vi "test_read-nmea-data2.vi"() -> ()   [LabVIEW 2019] (continued)
F9P\t\t\n15:11:02.15\tF9P\t\t\n15:11:02.17\tF9P\t\t\n15:11:02.19\tF9P\t\t\n15:11:02.21\tF9P\t\t\n15:11:02.23\tF9P\t\t\n15:11:02.25\tF9P\t$GNRMC,061104.00,A,3723.54880,N,12656.89488,E,2.304,137.20,250720,,,A,V*0F\n\t\n15:11:02.27\tF9P\t$GNVTG,137.20,T,,M,2.304,N,4.267,K,A*26\n\t\n15:11:02.29\tF9P\t$GNGGA,061104.00,3723.54880,N,12656.89488,E,1,12,0.68,63.8,M,18.5,M,,*7B\n\t\n15:11:02.31\tF9P\t$GNGSA,A,3,12,06,19,05,17,09,02,,,,,,1.28,0.68,1.08,1*08\n\t\n15:11:02.33\tF9P\t$GNGSA,A,3,85,71,84,,,,,,,,,,1.28,0.68,1.08,2*09\n\t\n15:11:02.35\tF9P\t$GNGSA,A,3,36,19,11,04,09,12,,,,,,,1.28,0.68,1.08,3*0C\n\t\n15:11:02.37\tF9P\t$GNGSA,A,3,14,11,33,,,,,,,,,,1.28,0.68,1.08,4*0D\n\t\n15:11:02.39\tF9P\t$GPGSV,3,1,09,02,54,318,32,04,18,044,,05,37,247,22,06,64,047,29,1*66\n\t\n15:11:02.41\tF9P\t$GPGSV,3,2,09,09,45,074,22,12,24,277,21,17,33,153,31,19,53,157,22,1*6D\n\t\n15:11:02.43\tF9P\t$GPGSV,3,3,09,25,12,307,,1*5D\n\t\n15:11:02.45\tF9P\t$GPGSV,3,1,09,02,54,318,,04,18,044,,05,37,247,,06,64,047,,6*6B\n\t\n15:11:02.47\tF9P\t$GPGSV,3,2,09,09,45,074,22,12,24,277,,17,33,153,13,19,53,157,,6*69\n\t\n15:11:02.49\tF9P\t$GPGSV,3,3,09,25,12,307,,6*5A\n\t\n15:11:02.51\tF9P\t$GLGSV,2,1,08,69,12,031,,70,72,041,,71,51,205,16,72,03,209,,1*75\n\t\n15:11:02.53\tF9P\t$GLGSV,2,2,08,77,01,326,,84,20,122,07,85,70,065,24,86,36,330,,1*7A\n\t\n15:11:02.55\tF9P\t$GLGSV,2,1,08,69,12,031,,70,72,041,,71,51,205,20,72,03,209,,3*72\n\t\n15:11:02.57\tF9P\t$GLGSV,2,2,08,77,01,326,,84,20,122,19,85,70,065,19,86,36,330,,3*79\n\t\n15:11:02.59\tF9P\t$GAGSV,2,1,08,02,08,297,10,04,66,118,24,09,31,193,18,11,71,357,20,7*79\n\t\n15:11:02.61\tF9P\t$GAGSV,2,2,08,12,40,102,19,19,27,045,09,25,09,249,,36,25,308,13,7*78\n\t\n15:11:02.63\tF9P\t$GAGSV,2,1,08,02,08,297,,04,66,118,25,09,31,193,,11,71,357,,2*77\n\t\n15:11:02.65\tF9P\t$GAGSV,2,2,08,12,40,102,27,19,27,045,,25,09,249,,36,25,308,,2*7B\n\t\n15:11:02.67\tF9P\t$GBGSV,1,1,03,11,50,131,19,14,87,138,20,33,60,219,22,1*45\n\t\n15:11:02.69\tF9P\t$GBGSV,1,1,03,11,50,131,29,14,87,138,21,33,60,219,,3*45\n\t\n15:11:02.71\tF9P\t$GNGLL,3723.54880,N,12656.89488,E,061104.00,A,A*72\n\t\n15:11:02.73\tF9P\t\t\n15:11:02.75\tF9P\t\t\n15:11:02.77\tF9P\t\t\n15:11:02.79\tF9P\t\t\n15:11:02.81\tF9P\t\t\n15:11:02.83\tF9P\t\t\n15:11:02.85\tF9P\t\t\n15:11:02.87\tF9P\t\t\n15:11:02.89\tF9P\t\t\n15:11:02.91\tF9P\t\t\n15:11:02.93\tF9P\t\t\n15:11:02.95\tF9P\t\t\n15:11:02.97\tF9P\t\t\n15:11:02.99\tF9P\t\t\n15:11:03.01\tF9P\t\t\n15:11:03.03\tF9P\t\t\n15:11:03.05\tF9P\t\t\n15:11:03.07\tF9P\t\t\n15:11:03.09\tF9P\t\t\n15:11:03.11\tF9P\t\t\n15:11:03.13\tF9P\t\t\n15:11:03.15\tF9P\t\t\n15:11:03.17\tF9P\t\t\n15:11:03.19\tF9P\t\t\n15:11:03.21\tF9P\t\t\n15:11:03.23\tF9P\t\t\n15:11:03.25\tF9P\t$GNRMC,061105.00,A,3723.54859,N,12656.89546,E,2.284,,250720,,,A,V*19\n\t\n15:11:03.27\tF9P\t$GNVTG,,T,,M,2.284,N,4.231,K,A*35\n\t\n15:11:03.29\tF9P\t$GNGGA,061105.00,3723.54859,N,12656.89546,E,1,12,0.69,62.1,M,18.5,M,,*74\n\t\n15:11:03.31\tF9P\t$GNGSA,A,3,12,06,19,05,17,09,02,,,,,,1.28,0.69,1.08,1*09\n\t\n15:11:03.33\tF9P\t$GNGSA,A,3,85,71,84,,,,,,,,,,1.28,0.69,1.08,2*08\n\t\n15:11:03.35\tF9P\t$GNGSA,A,3,36,19,11,04,09,12,,,,,,,1.28,0.69,1.08,3*0D\n\t\n15:11:03.37\tF9P\t$GNGSA,A,3,14,11,33,,,,,,,,,,1.28,0.69,1.08,4*0C\n\t\n15:11:03.39\tF9P\t$GPGSV,3,1,09,02,54,318,35,04,18,044,,05,37,247,23,06,64,047,24,1*6D\n\t\n15:11:03.41\tF9P\t$GPGSV,3,2,09,09,45,074,24,12,24,277,20,17,33,153,25,19,53,157,22,1*6F\n\t\n15:11:03.43\tF9P\t$GPGSV,3,3,09,25,12,307,,1*5D\n\t\n15:11:03.45\tF9P\t$GPGSV,3,1,09,02,54,318,,04,18,044,,05,37,247,,06,64,047,,6*6B\n\t\n15:11:03.47\tF9P\t$GPGSV,3,2,09,09,45,074,23,12,24,277,,17,33,153,17,19,53,157,,6*6C\n\t\n15:11:03.49\tF9P\t$GPGSV,3,3,09,25,12,307,,6*5A\n\t\n15:11:03.51\tF9P\t$GLGSV,2,1,08,69,12,031,,70,72,041,,71,51,205,16,72,03,209,,1*75\n\t\n15:11:03.53\tF9P\t$GLGSV,2,2,08,77,01,326,,84,20,122,10,85,70,065,24,86,36,330,,1*7C\n\t\n15:11:03.55\tF9P\t$GLGSV,2,1,08,69,12,031,,70,72,041,,71,51,205,20,72,03,209,,3*72\n\t\n15:11:03.57\tF9P\t$GLGSV,2,2,08,77,01,326,,84,20,122,20,85,70,065,19,86,36,330,,3*73\n\t\n15:11:03.59\tF9P\t$GAGSV,2,1,08,02,08,297,09,04,66,118,23,09,32,193,19,11,71,357,21,7*75\n\t\n15:11:03.61\tF9P\t$GAGSV,2,2,08,12,40,102,18,19,27,045,09,25,09,249,,36,25,308,15,7*7F\n\t\n15:11:03.63\tF9P\t$GAGSV,2,1,08,02,08,297,,04,66,118,24,09,32,193,,11,71,357,,2*75\n\t\n15:11:03.65\tF9P\t$GAGSV,2,2,08,12,40,102,26,19,27,045,,25,09,249,,36,25,308,,2*7A\n\t\n15:11:03.67\tF9P\t$GBGSV,1,1,03,11,50,131,18,14,87,138,22,33,60,219,22,1*46\n\t\n15:11:03.69\tF9P\t$GBGSV,1,1,03,11,50,131,25,14,87,138,21,33,60,219,,3*49\n\t\n15:11:03.71\tF9P\t$GNGLL,3723.54859,N,12656.89546,E,061105.00,A,A*74\n\t\n15:11:03.73\tF9P\t\t\n15:11:03.75\tF9P\t\t\n15:11:03.77\tF9P\t\t\n15:11:03.79\tF9P\t\t\n15:11:03.81\tF9P\t\t\n15:11:03.83\tF9P\t\t\n15:11:03.85\tF9P\t\t\n15:11:03.87\tF9P\t\t\n15:11:03.89\tF9P\t\t\n15:11:03.91\tF9P\t\t\n15:11:03.93\tF9P\t\t\n15:11:03.95\tF9P\t\t\n15:11:03.97\tF9P\t\t\n15:11:03.99\tF9P\t\t\n15:11:04.01\tF9P\t\t\n15:11:04.03\tF9P\t\t\n15:11:04.05\tF9P\t\t\n15:11:04.07\tF9P\t\t\n15:11:04.09\tF9P\t\t\n15:11:04.11\tF9P\t\t\n15:11:04.13\tF9P\t\t\n15:11:04.15\tF9P\t\t\n15:11:04.17\tF9P\t\t\n15:11:04.19\tF9P\t\t\n15:11:04.21\tF9P\t\t\n15:11:04.23\tF9P\t\t\n15:11:04.25\tF9P\t$GNRMC,061106.00,A,3723.54835,N,12656.89610,E,2.748,125.54,250720,,,A,V*0C\n\t\n15:11:04.27\tF9P\t$GNVTG,125.54,T,,M,2.748,N,5.089,K,A*29\n\t\n15:11:04.29\tF9P\t$GNGGA,061106.00,3723.54835,N,12656.89610,E,1,12,0.69,60.9,M,18.5,M,,*77\n\t\n15:11:04.31\tF9P\t$GNGSA,A,3,12,06,19,05,17,09,02,,,,,,1.28,0.69,1.08,1*09\n\t\n15:11:04.33\tF9P\t$GNGSA,A,3,85,71,84,,,,,,,,,,1.28,0.69,1.08,2*08\n\t\n15:11:04.35\tF9P\t$GNGSA,A,3,36,19,11,04,09,12,,,,,,,1.28,0.69,1.08,3*0D\n\t\n15:11:04.37\tF9P\t$GNGSA,A,3,14,11,33,,,,,,,,,,1.28,0.69,1.08,4*0C\n\t\n15:11:04.39\tF9P\t$GPGSV,3,1,09,02,54,318,36,04,18,044,,05,37,247,25,06,64,047,28,1*64\n\t\n15:11:04.41\tF9P\t$GPGSV,3,2,09,09,45,074,25,12,24,277,21,17,33,153,26,19,53,157,24,1*6A\n\t\n15:11:04.43\tF9P\t$GPGSV,3,3,09,25,12,307,,1*5D\n\t\n15:11:04.45\tF9P\t$GPGSV,3,1,09,02,54,318,,04,18,044,,05,37,247,,06,64,047,,6*6B\n\t\n15:11:04.47\tF9P\t$GPGSV,3,2,09,09,45,074,23,12,24,277,,17,33,153,18,19,53,157,,6*63\n\t\n15:11:04.49\tF9P\t$GPGSV,3,3,09,25,12,307,,6*5A\n\t\n15:11:04.51\tF9P\t$GLGSV,2,1,08,69,12,031,,70,72,041,,71,51,205,17,72,03,209,,1*74\n\t\n15:11:04.53\tF9P\t$GLGSV,2,2,08,77,01,326,,84,20,122,12,85,70,065,25,86,36,330,,1*7F\n\t\n15:11:04.55\tF9P\t$GLGSV,2,1,08,69,12,031,,70,72,041,,71,51,205,22,72,03,209,,3*70\n\t\n15:11:04.57\tF9P\t$GLGSV,2,2,08,77,01,326,,84,20,122,19,85,70,065,20,86,36,330,,3*73\n\t\n15:11:04.59\tF9P\t$GAGSV,2,1,08,02,08,297,07,04,66,118,25,09,32,193,18,11,71,358,22,7*70\n\t\n15:11:04.61\tF9P\t$GAGSV,2,2,08,12,40,102,18,19,27,045,11,25,09,249,,36,25,308,17,7*74\n\t\n15:11:04.63\tF9P\t$GAGSV,2,1,08,02,08,297,,04,66,118,23,09,32,193,,11,71,358,,2*7D\n\t\n15:11:04.65\tF9P\t$GAGSV,2,2,08,12,40,102,26,19,27,045,,25,09,249,,36,25,308,,2*7A\n\t\n15:11:04.67\tF9P\t$GBGSV,1,1,03,11,50,131,18,14,87,138,24,33,60,219,23,1*41\n\t\n15:11:04.69\tF9P\t$GBGSV,1,1,03,11,50,131,25,14,87,138,21,33,60,219,,3*49\n\t\n15:11:04.71\tF9P\t$GNGLL,3723.54835,N,12656.89610,E,061106.00,A,A*7D\n\t\n15:11:04.73\tF9P\t\t\n15:11:04.75\tF9P\t\t\n15:11:04.77\tF9P\t\t\n15:11:04.79\tF9P\t\t\n15:11:04.81\tF9P\t\t\n15:11:04.83\tF9P\t\t\n15:11:04.85\tF9P\t\t\n15:11:04.87\tF9P\t\t\n15:11:04.89\tF9P\t\t\n15:11:04.91\tF9P\t\t\n15:11:04.93\tF9P\t\t\n15:11:04.95\tF9P\t\t\n15:11:04.97\tF9P\t\t\n15:11:04.99\tF9P\t\t\n15:11:05.01\tF9P\t\t\n15:11:05.03\tF9P\t\t\n15:11:05.05\tF9P\t\t\n15:11:05.07\tF9P\t\t\n15:11:05.09\tF9P\t\t\n15:11:05.11\tF9P\t\t\n15:11:05.13\tF9P\t\t\n15:11:05.15\tF9P\t\t\n15:11:05.17\tF9P\t\t\n15:11:05.19\tF9P\t\t\n15:11:05.21\tF9P\t\t\n15:11:05.23\tF9P\t\t\n15:11:05.25\tF9P\t$GNRMC,061107.00,A,3723.54762,N,12656.89644,E,2.460,139.61,250720,,,A,V*03\n\t\n15:11:05.27\tF9P\t$GNVTG,139.61,T,,M,2.460,N,4.557,K,A*2C\n\t\n15:11:05.29\tF9P\t$GNGGA,061107.00,3723.54762,N,12656.89644,E,1,12,0.69,60.4,M,18.5,M,,*77\n\t\n15:11:05.31\tF9P\t$GNGSA,A,3,12,06,19,05,17,09,02,,,,,,1.28,0.69,1.08,1*09\n\t\n15:11:05.33\tF9P\t$GNGSA,A,3,85,71,84,,,,,,,,,,1.28,0.69,1.08,2*08\n\t\n15:11:05.35\tF9P\t$GNGSA,A,3,36,19,11,04,09,12,,,,,,,1.28,0.69,1.08,3*0D\n\t\n15:11:05.37\tF9P\t$GNGSA,A,3,14,11,33,,,,,,,,,,1.28,0.69,1.08,4*0C\n\t\n15:11:05.39\tF9P\t$GPGSV,3,1,09,02,54,318,28,04,18,044,,05,37,247,26,06,64,047,28,1*68\n\t\n15:11:05.41\tF9P\t$GPGSV,3,2,09,09,45,074,24,12,24,277,20,17,33,153,26,19,53,157,23,1*6D\n\t\n15:11:05.43\tF9P\t$GPGSV,3,3,09,25,12,307,,1*5D\n\t\n15:11:05.45\tF9P\t$GPGSV,3,1,09,02,54,318,,04,18,044,,05,37,247,,06,64,047,21,6*68\n\t\n15:11:05.47\tF9P\t$GPGSV,3,2,09,09,45,074,24,12,24,277,,17,33,153,18,19,53,157,,6*64\n\t\n15:11:05.49\tF9P\t$GPGSV,3,3,09,25,12,307,,6*5A\n\t\n15:11:05.51\tF9P\t$GLGSV,2,1,08,69,12,031,,70,72,041,,71,51,205,17,72,03,209,,1*74\n\t\n15:11:05.53\tF9P\t$GLGSV,2,2,08,77,01,326,,84,20,122,08,85,70,065,26,86,36,330,,1*77\n\t\n15:11:05.55\tF9P\t$GLGSV,2,1,08,69,12,031,,70,72,041,,71,51,205,21,72,03,209,,3*73\n\t\n15:11:05.57\tF9P\t$GLGSV,2,2,08,77,01,326,,84,20,122,20,85,70,065,21,86,36,330,,3*78\n\t\n15:11:05.59\tF9P\t$GAGSV,2,1,08,02,08,297,12,04,66,118,22,09,32,193,17,11,71,358,22,7*7C\n\t\n15:11:05.61\tF9P\t$GAGSV,2,2,08,12,40,102,17,19,27,045,13,25,09,249,,36,25,308,19,7*77\n\t\n15:11:05.63\tF9P\t$GAGSV,2,1,08,02,08,297,,04,66,118,21,09,32,193,,11,71,358,,2*7F\n\t\n15:11:05.65\tF9P\t$GAGSV,2,2,08,12,40,102,23,19,27,045,,25,09,249,,36,25,308,,2*7F\n\t\n15:11:05.67\tF9P\t$GBGSV,1,1,03,11,50,131,18,14,87,138,21,33,60,219,21,1*46\n\t\n15:11:05.69\tF9P\t$GBGSV,1,1,03,11,50,131,25,14,87,138,,33,60,219,,3*4A\n\t\n15:11:05.71\tF9P\t$GNGLL,3723.54762,N,12656.89644,E,061107.00,A,A*70\n\t\n15:11:05.73\tF9P\t\t\n15:11:05.75\tF9P\t\t\n15:11:05.77\tF9P\t\t\n15:11:05.79\tF9P\t\t\n15:11:05.81\tF9P\t\t\n15:11:05.83\tF9P\t\t\n15:11:05.85\tF9P\t\t\n15:11:05.87\tF9P\t\t\n15:11:05.89\tF9P\t\t\n15:11:05.91\tF9P\t\t\n15:11:05.93\tF9P\t\t\n15:11:05.95\tF9P\t\t\n15:11:05.97\tF9P\t\t\n15:11:05.99\tF9P\t\t\n15:11:06.01\tF9P\t\t\n15:11:06.03\tF9P\t\t\n15:11:06.05\tF9P\t\t\n15:11:06.07\tF9P\t\t\n15:11:06.09\tF9P\t\t\n15:11:06.11\tF9P\t\t\n15:11:06.13\tF9P\t\t\n15:11:06.15\tF9P\t\t\n15:11:06.17\tF9P\t\t\n15:11:06.19\tF9P\t\t\n15:11:06.21\tF9P\t\t\n15:11:06.23\tF9P\t\t\n15:11:06.25\tF9P\t$GNRMC,061108.00,A,3723.54695,N,12656.89698,E,3.008,136.67,250720,,,A,V*06\n\t\n15:11:06.27\tF9P\t$GNVTG,136.67,T,,M,3.008,N,5.572,K,A*28\n\t\n15:11:06.29\tF9P\t$GNGGA,061108.00,3723.54695,N,12656.89698,E,1,12,0.69,59.6,M,18.5,M,,*78\n\t\n15:11:06.31\tF9P\t$GNGSA,A,3,12,06,19,05,17,09,02,,,,,,1.28,0.69,1.08,1*09\n\t\n15:11:06.33\tF9P\t$GNGSA,A,3,85,71,84,,,,,,,,,,1.28,0.69,1.08,2*08\n\t\n15:11:06.35\tF9P\t$GNGSA,A,3,36,19,11,04,09,12,,,,,,,1.28,0.69,1.08,3*0D\n\t\n15:11:06.37\tF9P\t$GNGSA,A,3,14,11,33,,,,,,,,,,1.28,0.69,1.08,4*0C\n\t\n15:11:06.39\tF9P\t$GPGSV,3,1,09,02,54,318,34,04,18,044,15,05,37,247,25,06,64,047,30,1*6B\n\t\n15:11:06.41\tF9P\t$GPGSV,3,2,09,09,45,074,25,12,24,277,20,17,33,153,27,19,53,157,22,1*6C\n\t\n15:11:06.43\tF9P\t$GPGSV,3,3,09,25,12,307,,1*5D\n\t\n15:11:06.45\tF9P\t$GPGSV,3,1,09,02,54,318,,04,18,044,,05,37,247,20,06,64,047,21,6*6A\n\t\n15:11:06.47\tF9P\t$GPGSV,3,2,09,09,45,074,23,12,24,277,,17,33,153,18,19,53,157,,6*63\n\t\n15:11:06.49\tF9P\t$GPGSV,3,3,09,25,12,307,,6*5A\n\t\n15:11:06.51\tF9P\t$GLGSV,2,1,08,69,12,031,,70,72,041,,71,51,205,17,72,03,209,,1*74\n\t\n15:11:06.54\tF9P\t$GLGSV,2,2,08,77,01,326,,84,20,122,09,85,70,065,27,86,36,330,,1*77\n\t\n15:11:06.56\tF9P\t$GLGSV,2,1,08,69,12,031,,70,72,041,,71,51,205,21,72,03,209,,3*73\n\t\n15:11:06.58\tF9P\t$GLGSV,2,2,08,77,01,326,,84,20,122,19,85,70,065,23,86,36,330,,3*70\n\t\n15:11:06.60\tF9P\t$GAGSV,2,1,08,02,08,297,09,04,66,118,21,09,32,193,16,11,71,358,23,7*75\n\t\n15:11:06.62\tF9P\t$GAGSV,2,2,08,12,40,102,17,19,27,045,09,25,09,249,,36,25,308,18,7*7D\n\t\n15:11:06.64\tF9P\t$GAGSV,2,1,08,02,08,297,,04,66,118,23,09,32,193,,11,71,358,,2*7D\n\t\n15:11:06.66\tF9P\t$GAGSV,2,2,08,12,40,102,23,19,27,045,,25,09,249,,36,25,308,,2*7F\n\t\n15:11:06.68\tF9P\t$GBGSV,1,1,03,11,50,131,19,14,87,138,21,33,60,219,19,1*4C\n\t\n15:11:06.70\tF9P\t$GBGSV,1,1,03,11,50,131,31,14,87,138,,33,60,219,,3*4F\n\t\n15:11:06.72\tF9P\t$GNGLL,3723.54695,N,12656.89698,E,061108.00,A,A*77\n\t\n15:11:06.74\tF9P\t\t\n15:11:06.76\tF9P\t\t\n15:11:06.78\tF9P\t\t\n15:11:06.80\tF9P\t\t\n15:11:06.82\tF9P\t\t\n15:11:06.84\tF9P\t\t\n15:11:06.86\tF9P\t\t\n15:11:06.88\tF9P\t\t\n15:11:06.90\tF9P\t\t\n15:11:06.92\tF9P\t\t\n15:11:06.94\tF9P\t\t\n15:11:06.96\tF9P\t\t\n15:11:06.98\tF9P\t\t\n15:11:07.00\tF9P\t\t\n15:11:07.02\tF9P\t\t\n15:11:07.04\tF9P\t\t\n15:11:07.06\tF9P\t\t\n15:11:07.08\tF9P\t\t\n15:11:07.10\tF9P\t\t\n15:11:07.12\tF9P\t\t\n15:11:07.14\tF9P\t\t\n15:11:07.16\tF9P\t\t\n15:11:07.18\tF9P\t\t\n15:11:07.20\tF9P\t\t\n15:11:07.22\tF9P\t\t\n15:11:07.24\tF9P\t$GNRMC,061109.00,A,3723.54621,N,12656.89731,E,2.411,142.02,250720,,,A,V*07\n\t\n15:11:07.26\tF9P\t$GNVTG,142.02,T,,M,2.411,N,4.465,K,A*23\n\t\n15:11:07.28\tF9P\t$GNGGA,061109.00,3723.54621,N,12656.89731,E,1,12,0.69,60.1,M,18.5,M,,*79\n\t\n15:11:07.30\tF9P\t$GNGSA,A,3,12,06,19,05,17,09,02,,,,,,1.28,0.69,1.08,1*09\n\t\n15:11:07.32\tF9P\t$GNGSA,A,3,85,71,84,,,,,,,,,,1.28,0.69,1.08,2*08\n\t\n15:11:07.34\tF9P\t$GNGSA,A,3,36,19,11,04,09,12,,,,,,,1.28,0.69,1.08,3*0D\n\t\n15:11:07.36\tF9P\t$GNGSA,A,3,14,11,33,,,,,,,,,,1.28,0.69,1.08,4*0C\n\t\n15:11:07.38\tF9P\t$GPGSV,3,1,09,02,54,318,35,04,18,044,13,05,37,247,25,06,64,047,29,1*64\n\t\n15:11:07.40\tF9P\t$GPGSV,3,2,09,09,45,074,26,12,24,277,20,17,33,153,25,19,53,157,24,1*6B\n\t\n15:11:07.42\tF9P\t$GPGSV,3,3,09,25,12,307,,1*5D\n\t\n15:11:07.44\tF9P\t$GPGSV,3,1,09,02,54,318,,04,18,044,,05,37,247,17,06,64,047,20,6*6F\n\t\n15:11:07.46\tF9P\t$GPGSV,3,2,09,09,45,074,22,12,24,277,,17,33,153,18,19,53,157,,6*62\n\t\n15:11:07.48\tF9P\t$GPGSV,3,3,09,25,12,307,,6*5A\n\t\n15:11:07.50\tF9P\t$GLGSV,2,1,08,69,12,031,,70,72,041,,71,51,205,17,72,03,209,,1*74\n\t\n15:11:07.52\tF9P\t$GLGSV,2,2,08,77,01,326,,84,20,122,09,85,70,065,25,86,36,330,,1*75\n\t\n15:11:07.54\tF9P\t$GLGSV,2,1,08,69,12,031,,70,72,041,,71,51,205,20,72,03,209,,3*72\n\t\n15:11:07.56\tF9P\t$GLGSV,2,2,08,77,01,326,,84,20,122,19,85,70,065,24,86,36,330,,3*77\n\t\n15:11:07.58\tF9P\t$GAGSV,2,1,08,02,08,297,11,04,66,118,21,09,32,193,17,11,71,358,23,7*7D\n\t\n15:11:07.60\tF9P\t$GAGSV,2,2,08,12,40,102,17,19,27,045,10,25,09,249,,36,25,308,21,7*7F\n\t\n15:11:07.62\tF9P\t$GAGSV,2,1,08,02,08,297,,04,66,118,23,09,32,193,,11,71,358,,2*7D\n\t\n15:11:07.64\tF9P\t$GAGSV,2,2,08,12,40,102,21,19,27,045,,25,09,249,,36,25,308,,2*7D\n\t\n15:11:07.66\tF9P\t$GBGSV,1,1,03,11,50,131,19,14,87,138,21,33,60,219,19,1*4C\n\t\n15:11:07.68\tF9P\t$GBGSV,1,1,03,11,50,131,33,14,87,138,21,33,60,219,,3*4E\n\t\n15:11:07.70\tF9P\t$GNGLL,3723.54621,N,12656.89731,E,061109.00,A,A*7B\n\t\n15:11:07.72\tF9P\t\t\n15:11:07.74\tF9P\t\t\n15:11:07.76\tF9P\t\t\n15:11:07.78\tF9P\t\t\n15:11:07.80\tF9P\t\t\n15:11:07.82\tF9P\t\t\n15:11:07.84\tF9P\t\t\n15:11:07.86\tF9P\t\t\n15:11:07.88\tF9P\t\t\n15:11:07.90\tF9P\t\t\n15:11:07.92\tF9P\t\t\n15:11:07.94\tF9P\t\t\n15:11:07.96\tF9P\t\t\n15:11:07.98\tF9P\t\t\n15:11:08.00\tF9P\t\t\n15:11:08.02\tF9P\t\t\n15:11:08.04\tF9P\t\t\n15:11:08.06\tF9P\t\t\n15:11:08.08\tF9P\t\t\n15:11:08.10\tF9P\t\t\n15:11:08.12\tF9P\t\t\n15:11:08.14\tF9P\t\t\n15:11:08.16\tF9P\t\t\n15:11:08.18\tF9P\t\t\n15:11:08.20\tF9P\t\t\n15:11:08.22\tF9P\t\t\n15:11:08.24\tF9P\t$GNRMC,061110.00,A,3723.54616,N,12656.89727,E,1.799,133.01,250720,,,A,V*09\n\t\n15:11:08.26\tF9P\t$GNVTG,133.01,T,,M,1.799,N,3.332,K,A*24\n\t\n15:11:08.28\tF9P\t$GNGGA,061110.00,3723.54616,N,12656.89727,E,1,12,0.76,59.4,M,18.5,M,,*73\n\t\n15:11:08.30\tF9P\t$GNGSA,A,3,12,06,19,05,17,09,02,,,,,,1.40,0.76,1.18,1*08\n\t\n15:11:08.32\tF9P\t$GNGSA,A,3,85,71,84,,,,,,,,,,1.40,0.76,1.18,2*09\n\t\n15:11:08.34\tF9P\t$GNGSA,A,3,36,19,11,04,09,12,,,,,,,1.40,0.76,1.18,3*0C\n\t\n15:11:08.36\tF9P\t$GNGSA,A,3,14,11,33,,,,,,,,,,1.40,0.76,1.18,4*0D\n\t\n15:11:08.38\tF9P\t$GPGSV,3,1,09,02,54,318,44,04,18,044,,05,37,247,27,06,64,047,40,1*6D\n\t\n15:11:08.40\tF9P\t$GPGSV,3,2,09,09,45,074,25,12,24,277,22,17,33,153,31,19,53,157,34,1*6E\n\t\n15:11:08.42\tF9P\t$GPGSV,3,3,09,25,12,307,,1*5D\n\t\n15:11:08.44\tF9P\t$GPGSV,3,1,09,02,54,318,,04,18,044,,05,37,247,14,06,64,047,19,6*66\n\t\n15:11:08.46\tF9P\t$GPGSV,3,2,09,09,45,074,22,12,24,277,,17,33,153,20,19,53,157,,6*69\n\t\n15:11:08.48\tF9P\t$GPGSV,3,3,09,25,12,307,,6*5A\n\t\n15:11:08.50\tF9P\t$GLGSV,2,1,08,69,12,031,,70,72,041,,71,51,205,18,72,03,209,,1*7B\n\t\n15:11:08.52\tF9P\t$GLGSV,2,2,08,77,01,326,,84,20,122,08,85,70,065,31,86,36,330,,1*71\n\t\n15:11:08.54\tF9P\t$GLGSV,2,1,08,69,12,031,,70,72,041,,71,51,205,21,72,03,209,,3*73\n\t\n15:11:08.56\tF9P\t$GLGSV,2,2,08,77,01,326,,84,20,122,17,85,70,065,22,86,36,330,,3*7F\n\t\n15:11:08.58\tF9P\t$GAGSV,2,1,08,02,08,297,11,04,66,118,22,09,32,193,26,11,71,358,30,7*7E\n\t\n15:11:08.60\tF9P\t$GAGSV,2,2,08,12,40,102,18,19,26,045,10,25,09,249,,36,25,308,30,7*71\n\t\n15:11:08.62\tF9P\t$GAGSV,2,1,08,02,08,297,,04,66,118,24,09,32,193,,11,71,358,,2*7A\n\t\n15:11:08.64\tF9P\t$GAGSV,2,2,08,12,40,102,18,19,26,045,,25,09,249,,36,25,308,,2*76\n\t\n15:11:08.66\tF9P\t$GBGSV,1,1,03,11,50,131,21,14,87,138,25,33,60,219,23,1*4A\n\t\n15:11:08.68\tF9P\t$GBGSV,1,1,03,11,50,131,33,14,87,138,28,33,60,219,,3*47\n\t\n15:11:08.70\tF9P\t$GNGLL,3723.54616,N,12656.89727,E,061110.00,A,A*70\n\t\n15:11:08.72\tF9P\t\t\n15:11:08.74\tF9P\t\t\n15:11:08.76\tF9P\t\t\n15:11:08.78\tF9P\t\t\n15:11:08.80\tF9P\t\t\n15:11:08.82\tF9P\t\t\n15:11:08.84\tF9P\t\t\n15:11:08.86\tF9P\t\t\n15:11:08.88\tF9P\t\t\n15:11:08.90\tF9P\t\t\n15:11:08.92\tF9P\t\t\n15:11:08.94\tF9P\t\t\n15:11:08.96\tF9P\t\t\n15:11:08.98\tF9P\t\t\n15:11:09.00\tF9P\t\t\n15:11:09.02\tF9P\t\t\n15:11:09.04\tF9P\t\t\n15:11:09.06\tF9P\t\t\n15:11:09.08\tF9P\t\t\n15:11:09.10\tF9P\t\t\n15:11:09.12\tF9P\t\t\n15:11:09.14\tF9P\t\t\n15:11:09.16\tF9P\t\t\n15:11:09.18\tF9P\t\t\n15:11:09.20\tF9P\t\t\n15:11:09.22\tF9P\t\t\n15:11:09.24\tF9P\t$GNRMC,061111.00,A,3723.54534,N,12656.89756,E,1.880,139.63,25072\t\n15:11:09.26\tF9P\t0,,,A,V*04\n\t\n15:11:09.28\tF9P\t$GNVTG,139.63,T,,M,1.880,N,3.482,K,A*21\n\t\n15:11:09.30\tF9P\t$GNGGA,061111.00,3723.54534,N,12656.89756,E,1,12,0.68,57.4,M,18.5,M,,*76\n\t\n15:11:09.32\tF9P\t$GNGSA,A,3,12,06,19,05,17,09,02,,,,,,1.27,0.68,1.08,1*07\n\t\n15:11:09.34\tF9P\t$GNGSA,A,3,85,71,84,,,,,,,,,,1.27,0.68,1.08,2*06\n\t\n15:11:09.36\tF9P\t$GNGSA,A,3,36,19,11,04,09,12,,,,,,,1.27,0.68,1.08,3*03\n\t\n15:11:09.38\tF9P\t$GNGSA,A,3,14,11,33,,,,,,,,,,1.27,0.68,1.08,4*02\n\t\n15:11:09.40\tF9P\t$GPGSV,3,1,09,02,54,318,44,04,18,044,,05,37,247,25,06,64,047,31,1*69\n\t\n15:11:09.42\tF9P\t$GPGSV,3,2,09,09,45,074,28,12,24,277,30,17,33,153,36,19,53,157,30,1*63\n\t\n15:11:09.44\tF9P\t$GPGSV,3,3,09,25,12,307,,1*5D\n\t\n15:11:09.46\tF9P\t$GPGSV,3,1,09,02,54,318,,04,18,044,,05,37,247,14,06,64,047,17,6*68\n\t\n15:11:09.48\tF9P\t$GPGSV,3,2,09,09,45,074,20,12,24,277,,17,33,153,19,19,53,157,,6*61\n\t\n15:11:09.50\tF9P\t$GPGSV,3,3,09,25,12,307,,6*5A\n\t\n15:11:09.52\tF9P\t$GLGSV,2,1,08,69,12,031,,70,72,041,,71,51,205,20,72,03,209,,1*70\n\t\n15:11:09.54\tF9P\t$GLGSV,2,2,08,77,01,326,,84,20,122,16,85,70,065,25,86,36,330,,1*7B\n\t\n15:11:09.56\tF9P\t$GLGSV,2,1,08,69,12,031,,70,72,041,,71,51,205,20,72,03,209,,3*72\n\t\n15:11:09.58\tF9P\t$GLGSV,2,2,08,77,01,326,,84,20,122,16,85,70,065,21,86,36,330,,3*7D\n\t\n15:11:09.60\tF9P\t$GAGSV,2,1,08,02,08,297,10,04,66,118,30,09,32,193,21,11,71,358,25,7*7F\n\t\n15:11:09.62\tF9P\t$GAGSV,2,2,08,12,40,102,19,19,26,045,11,25,09,249,,36,25,308,21,7*71\n\t\n15:11:09.64\tF9P\t$GAGSV,2,1,08,02,08,297,,04,66,118,25,09,32,193,,11,71,358,,2*7B\n\t\n15:11:09.66\tF9P\t$GAGSV,2,2,08,12,40,102,19,19,26,045,,25,09,249,,36,25,308,,2*77\n\t\n15:11:09.68\tF9P\t$GBGSV,1,1,03,11,50,131,28,14,87,138,28,33,60,219,21,1*4C\n\t\n15:11:09.70\tF9P\t$GBGSV,1,1,03,11,50,131,29,14,87,138,25,33,60,219,,3*41\n\t\n15:11:09.72\tF9P\t$GNGLL,3723.54534,N,12656.89756,E,061111.00,A,A*74\n\t\n15:11:09.74\tF9P\t\t\n15:11:09.76\t
